vi "SetThreshold.vi"(8 "error in (no error)":errorcluster, 10 "Severity":T1=enum."INFO", 11 "LogManager in":refnum<class "LogManager.lvclass">) -> (0 "error out":errorcluster, 3 "LogManager out":refnum<class "LogManager.lvclass">)   [LabVIEW 2026, in "Lumberjack.lvlib" / "LogManager.lvclass"]
doc: "Updates the manager's stored global threshold.\nWrites the new Severity into the manager's resolved configuration so the next PostSnapshot publishes it as globalThreshold; the SetGlobalThresholdMsg:Do handler calls this and then re-posts the Snapshot.\nLumberjack.lvlib, LogManager.lvclass, public."
uses:
  LogManager.lvclass
  TypeDefs/Severity.ctl
  LogManager.lvclass/LogManager.ctl
  Lumberjack.lvlib
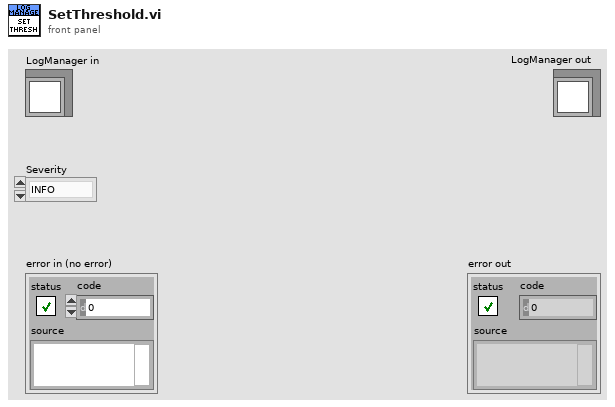
[diagram p1: front panel]
types:
  T1 = typedef "Lumberjack.lvlib/Severity.ctl" = enum16{"OFF", "FATAL", "ERROR", "WARN", "INFO", "DEBUG", "TRACE", "ALL"}
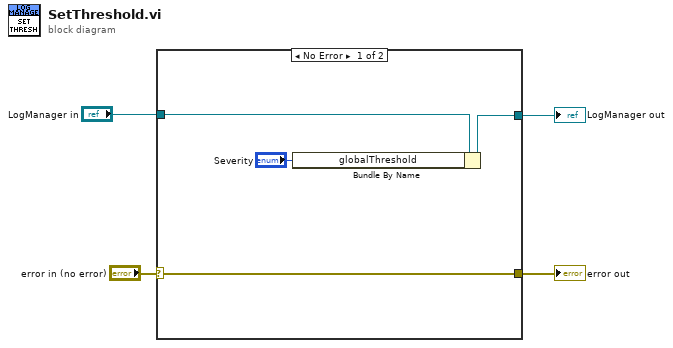
[diagram p0: block diagram]
diagram:
  n1 = case shown="No Error" "error in (no error)" {
    selector: "error in (no error)" -> [w5 w9]
    tunnel: "LogManager in" -> [w8 w10]
    tunnel: [w7 w10] -> w3
    tunnel: [w5 w9] -> w1
    frame No Error {
      n2 = Bundle By Name(cluster=w8, "globalThreshold"="Severity") -> (w7:refnum<class "LogManager.lvclass">)
    }
    frame Error {
    }
  }
  "error out" <- w1
  "LogManager out" <- w3
